vi "Execute.vi"(7 "Actor in":refnum<class "Actor.lvclass">, 8 "Error in":errorcluster, 11 "Stop Msg in":refnum<class "Stop Msg.lvclass">) -> (0 "Error out":errorcluster, 2 "Msg Output":refnum<class "Msg Output.lvclass">, 5 "Actor out":refnum<class "Actor.lvclass">)   [LabVIEW 2025, in "jettl.lvlib" / "Stop jettl Msg.lvlib" / "Stop Msg.lvlib" / "Stop Msg.lvclass"]
uses:
  Stop Msg.lvclass
  Actor/Actor.lvclass
  Msg Output/Msg Output.lvclass
  Stop jettl Msg/Stop jettl Msg.lvclass
  Stop Msg.lvclass/Stop Msg.ctl
  Stop Msg Input/Stop Msg Input.lvlib
  Stop Msg Output/Stop Msg Output.lvlib
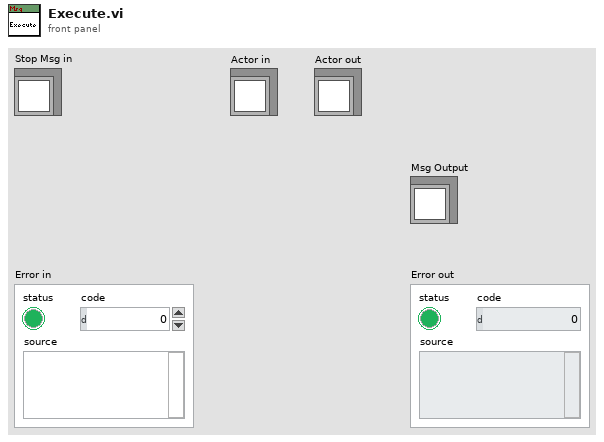
[diagram p1: front panel]
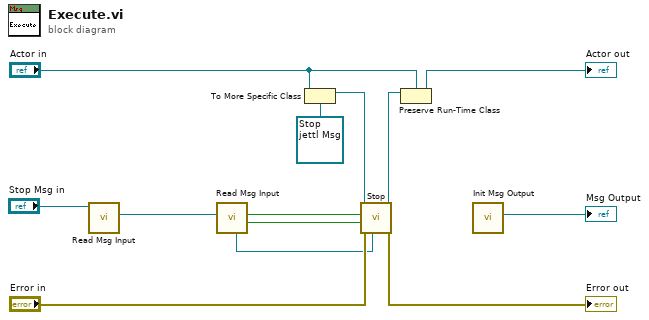
[diagram p0: block diagram]
diagram:
  n1 = call-dynamic "Read Msg Input.vi"("Stop Msg in"="Stop Msg in") -> ("Msg Input"=w5:refnum<class "Msg Input.lvclass">)  [unwired: 10 in]
  n2 = call "Read Msg Input.vi"("Msg Input"=w5) -> ("Parent Stopped"=w1:bool, "Safe Stop"=w2:bool, "Teller"=w4:refnum<class "Teller.lvclass">)  [unwired: 8 in]
  n3 = To More Specific Class(target class=refnum<class "Stop jettl Msg.lvclass"> refnum ("jettl.lvlib:Stop jettl Msg.lvlib:Stop jettl Msg.lvclass"), reference="Actor in") -> (specific class reference=w11:refnum<class "Stop jettl Msg.lvclass">)  [unwired: 1 in, 1 out]
  n4 = call-dynamic "Stop.vi"("Teller"=w4, "Error in"="Error in", "Parent Stopped"=w1, "Safe Stop"=w2, "Stop jettl Msg in"=w11) -> ("Error out"=→"Error out":errorcluster, "Stop jettl Msg out"=w10:refnum<class "Stop jettl Msg.lvclass">)  [unwired: 5 in]
  n5 = Preserve Run-Time Class(object in=w10, 2:"Actor in") -> (object out=→"Actor out":refnum<class "Actor.lvclass">)  [unwired: 1 in, 1 out]
  n6 = call "Init Msg Output.vi"() -> ("Msg Output"=→"Msg Output":refnum<class "Msg Output.lvclass">)  [unwired: 11 in]
